vi "Get QueueElements.vi"(8 "error in (no error)":errorcluster, 11 "PriorityQueue in":refnum<class "PriorityQueue.lvclass">) -> (0 "error out":errorcluster, 2 "Queue Elements":variant[](array[variant]), 3 "PriorityQueue out":refnum<class "PriorityQueue.lvclass">)   [LabVIEW 2019, in "PriorityQueue.lvclass"]
uses:
  PriorityQueue.lvclass
  PriorityQueue.lvclass/PriorityQueue.ctl
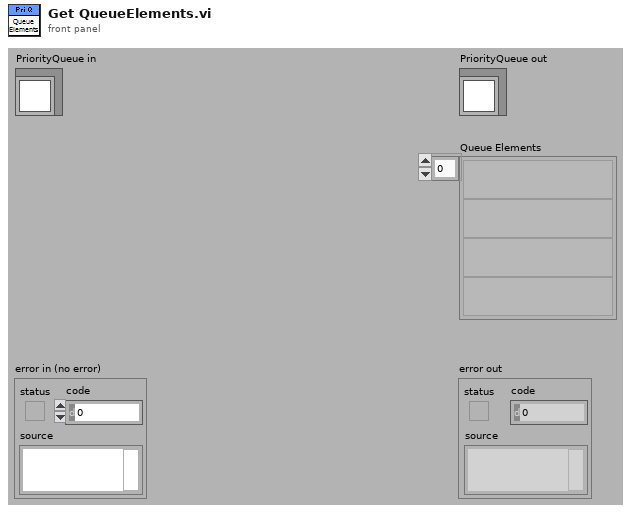
[diagram p1: front panel]
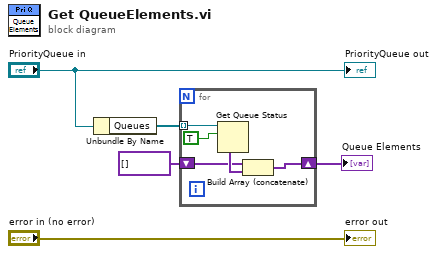
[diagram p0: block diagram]
diagram:
  n1 = Unbundle By Name("PriorityQueue in") -> ("Queues"=w5:refnum<queue>[])
  n2 = for {
    tunnel: w5 -> [w10] mode=indexing
    shift-right: [w7] -> w2
    shift-left: variant[] [] -> [w6]
    n3 = Get Queue Status(queue=w10, return elements? (F)=TRUE) -> (elements=w8:variant[])  [unwired: 1 in, 7 out]
    n4 = Build Array (concatenate)(w6, w8) -> (w7:variant[])
  }
  "Queue Elements" <- w2
  "error out" <- "error in (no error)"
  "PriorityQueue out" <- "PriorityQueue in"
